vi "CreateHTML.vi"(0 "reference in":refnum<class "Control.lvclass">, 2 "VI Name":string, 5 "error in (no error)":errorcluster) -> (13 "script dependencies":string[](array[string]), 14 "reference out":refnum<class "Control.lvclass">, 15 "HTML":string, 16 "js variables":string, 17 "js code for controls":string, 18 "js code for indicators":string, 19 "error out":errorcluster)   [LabVIEW 2014, in "Control.lvclass"]
uses:
  Control.lvclass
  Object_class/Object.lvclass
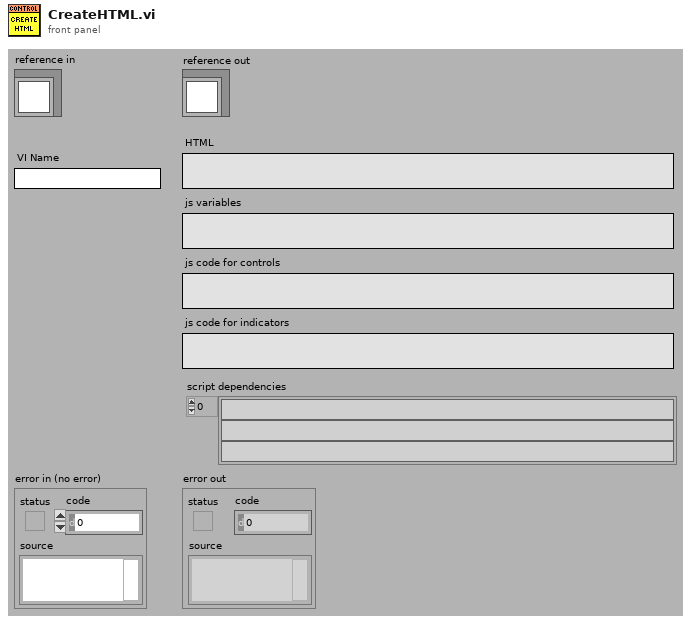
[diagram p1: front panel]
types:
  T1 = typedef "Object.lvclass/Attributes.ctl" = cluster{"UID":i32, "Type":string, "Coordinates":T2}
  T2 = typedef "Object.lvclass/Coordinates.ctl" = cluster{"Left":i32, "Top":i32, "Height":u32, "Width":u32}
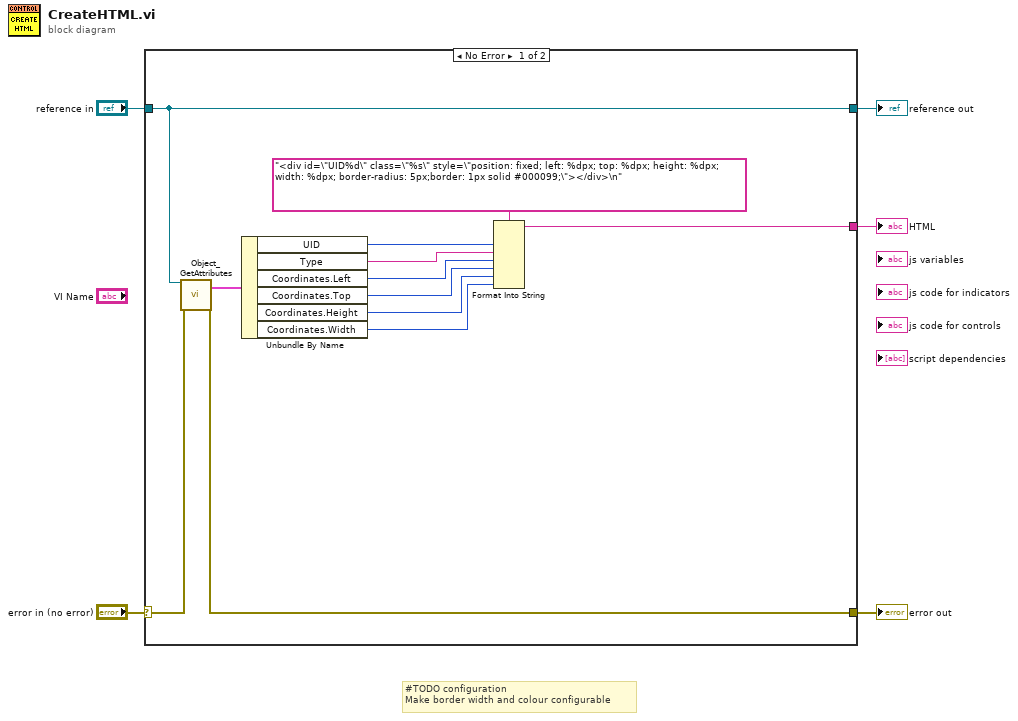
[diagram p0: block diagram]
diagram:
  # "#TODO configuration\nMake border width and colour configurable"
  n1 = case shown="No Error" "error in (no error)" {
    selector: "error in (no error)" -> [w6 w19]
    tunnel: [w8 w19] -> w4
    tunnel: [w7 w18] -> w2
    tunnel: "reference in" -> [w7 w18]
    tunnel: [w10 _] -> w1
    frame No Error {
      n2 = call "Object_GetAttributes.vi"("reference in"=w7, "error in (no error)"=w6) -> ("Data"=w9:T1, "error out"=w8:errorcluster)  [unwired: 14 in, 2 out]
      n3 = Unbundle By Name(w9) -> ("UID"=w16:i32, "Type"=w15:string, "Coordinates.Left"=w14:i32, "Coordinates.Top"=w13:i32, "Coordinates.Height"=w12:u32, "Coordinates.Width"=w11:u32)
      n4 = Format Into String(format string="<div id=\"UID%d\" class=\"%s\" style=\"position: fixed; left: %dpx; top: %dpx; height: %dpx; width: %dpx; border-radius: 5px;border: 1px solid #000099;\"></div>\n", w16, w15, w14, w13, w12, w11) -> (resulting string=w10:string)  [unwired: 2 in, 1 out]
    }
    frame Error {
    }
  }
  "error out" <- w4
  "reference out" <- w2
  "HTML" <- w1
